vi "CompressedEncryptedFileDataSource_Create.vi"(8 "error in (no error)":errorcluster, 9 "CompressionType(Type1)":T1, 10 "Name":string, 11 "reference in":refnum<class "CompressedEncryptedFileDataSource.lvclass">) -> (0 "error out":errorcluster, 3 "reference out":refnum<class "CompressedEncryptedFileDataSource.lvclass">)   [LabVIEW 2020, in "CompressedEncryptedFileDataSource.lvclass"]
uses:
  CompressedEncryptedFileDataSource.lvclass
  C:/Projects/OpenGDS_DesignPatterns/Decorator3/EncryptedFileDataSource_class/EncryptedFileDataSource.lvclass
  EncryptionType.ctl
  EncryptedFileDataSource_class/EncryptedFileDataSource.lvclass
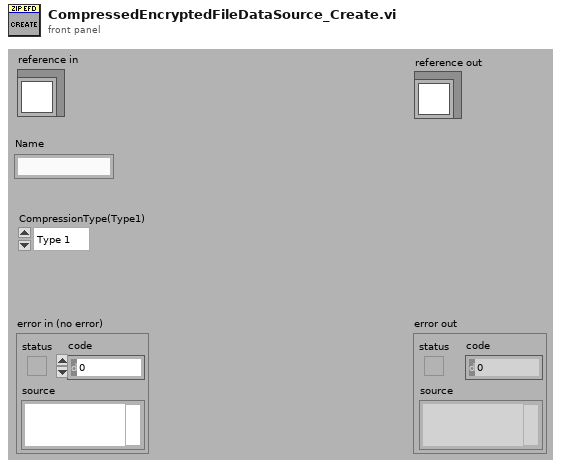
[diagram p1: front panel]
types:
  T1 = typedef "CompressedEncryptedFileDataSource.lvclass/EncryptionType.ctl" = enum16{"Type 1", "Type 2"}
  T2 = typedef "CompressedEncryptedFileDataSource.lvclass/ObjectAttributes.ctl" = cluster{"CompressionType":T1}
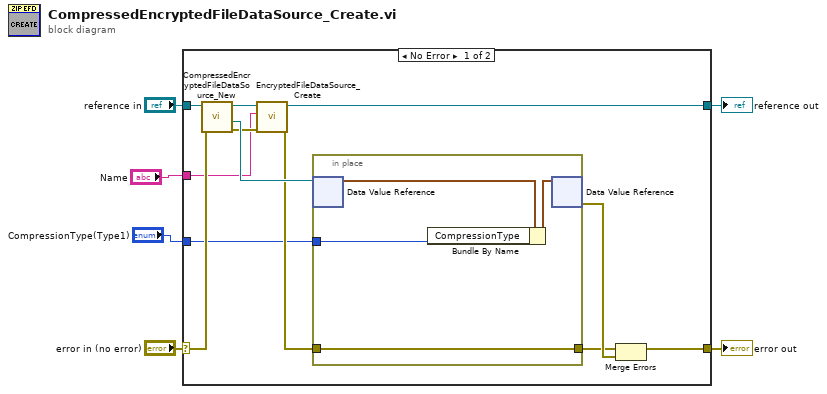
[diagram p0: block diagram]
diagram:
  n1 = case shown="No Error" "error in (no error)" {
    selector: "error in (no error)" -> [w14 w24]
    tunnel: [w12 w24] -> w5
    tunnel: "reference in" -> [w16 w23]
    tunnel: [w11 w23] -> w3
    tunnel: "Name" -> [w8 _]
    tunnel: "CompressionType(Type1)" -> [w7 _]
    frame No Error {
      n2 = call "CompressedEncryptedFileDataSource_New.vi"("error in (no error)"=w14, "reference in"=w16) -> ("error out"=w15:errorcluster, "DVRRefOut"=w18:refnum<data-value>, "reference out"=w17:refnum<class "CompressedEncryptedFileDataSource.lvclass">)  [unwired: 6 in, 1 out]
      n3 = call "EncryptedFileDataSource_Create.vi"("error in (no error)"=w15, "Name"=w8, "reference in"=w17) -> ("error out"=w10:errorcluster, "reference out"=w11:refnum<class "CompressedEncryptedFileDataSource.lvclass">)  [unwired: 7 in]
      n4 = in-place {
        in-place-border: w10 -> [w20]
        in-place-border: [w20] -> w9
        in-place-border: w7 -> [w19]
        n5 = in-place-dvr #1(w18) -> (w21:T2)  [unwired: 1 out]
        n6 = Bundle By Name(cluster=w21, "CompressionType"=w19) -> (w22:T2)
        n7 = in-place-dvr #1(w22) -> (w13:errorcluster)  [unwired: 1 out]
      }
      n8 = Merge Errors(w9, w13) -> (w12:errorcluster)
    }
    frame Error {
    }
  }
  "error out" <- w5
  "reference out" <- w3
